vi "AutoThresholdLocalization-4.vi"(4 "[IN] Gauss Filter":bool, 5 "[IN] Method":i32(ring) items=["clustering", "entropy", "metric", "moments", "inter-class variance"], 6 "[IN] Autothreshold Images \nInstead Of Generated U8":bool, 7 "[IN] Median Filter":bool, 8 "error IN":errorcluster, 10 "[IN] Binarized Image":T3, 11 "[IN] Source Image":T3) -> (0 "error OUT":errorcluster, 2 "[OUT] X,Y Coordinates":dbl[](array[numeric]))   [LabVIEW 2020]
uses:
  <vilib>/vision/Image Controls.llb/IMAQ Image.ctl
  <vilib>/vision/Image Controls.llb/IMAQ Rounding Mode.ctl
  <vilib>/vision/NI_Vision_Development_Module.lvlib
panel:
  in  "Selection Values":T2(array[cluster])=[{"Measurement Parameter"=22, "Range Lower Value"=10.0, "Range Upper Value"=800.0, "Range"=FALSE, "Measurement Type"=FALSE}] {"Measurement Parameter" items=["Center of Mass X", "Center of Mass Y", "First Pixel X", "First Pixel Y", "Bounding Rect Left", "Bounding Rect Top", "Bounding Rect Right", "Bounding Rect Bottom", "Max Feret Diameter Start X", "Max Feret Diameter Start Y", "Max Feret Diameter End X", "Max Feret Diameter End Y", "Max Horiz. Segment Length Left", "Max Horiz. Segment Length Right", "Max Horiz. Segment Length Row", "-", "Bounding Rect Width", "Bounding Rect Height", "Bounding Rect Diagonal", "Perimeter", "Convex Hull Perimeter", "Holes' Perimeter", "Max Feret Diameter", "Equivalent Ellipse Major Axis", "Equivalent Ellipse Minor Axis", "Equivalent Ellipse Minor Axis (Feret)", "Equivalent Rect Long Side", "Equivalent Rect Short Side", "Equivalent Rect Diagonal", "Equivalent Rect Short Side (Feret)", "Average Horiz. Segment Length", "Average Vert. Segment Length", "Hydraulic Radius", "Waddel Disk Diameter", "-", "Area", "Holes' Area", "Particle & Holes' Area", "Convex Hull Area", "Image Area", "-", "Number of Holes", "Number of Horiz. Segments", "Number of Vert. Segments", "-", "Orientation", "Max Feret Diameter Orientation", "-", "% Area/Image Area", "% Area/(Particle & Holes' Area)", "Ratio of Equivalent Ellipse Axes", "Ratio of Equivalent Rect Sides", "-", "Elongation Factor", "Compactness Factor", "Heywood Circularity Factor", "Type Factor", "-", "Sum X", "Sum Y", "Sum XX", "Sum XY", "Sum YY", "Sum XXX", "Sum XXY", "Sum XYY", "Sum YYY", "-", "Moment of Inertia XX", "Moment of Inertia XY", "Moment of Inertia YY", "Moment of Inertia XXX", "Moment of Inertia XXY", "Moment of Inertia XYY", "Moment of Inertia YYY", "Norm. Moment of Inertia XX", "Norm. Moment of Inertia XY", "Norm. Moment of Inertia YY", "Norm. Moment of Inertia XXX", "Norm. Moment of Inertia XXY", "Norm. Moment of Inertia XYY", "Norm. Moment of Inertia YYY", "Hu Moment 1", "Hu Moment 2", "Hu Moment 3", "Hu Moment 4", "Hu Moment 5", "Hu Moment 6", "Hu Moment 7"]}
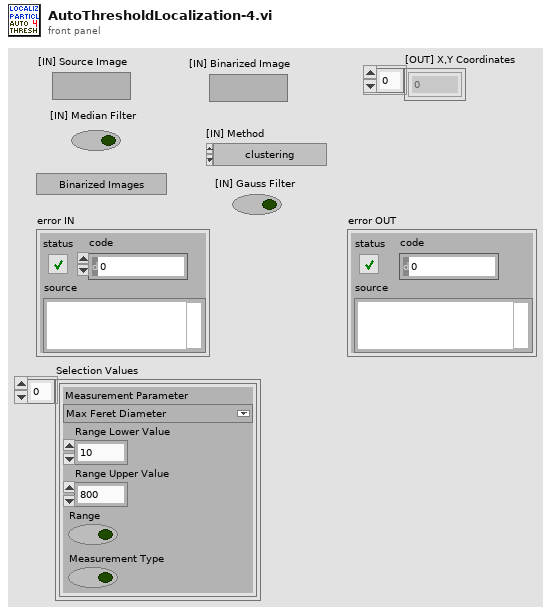
[diagram p1: front panel]
types:
  T1 = typedef "Particle Parameters" = i32
  T2 = cluster{"Measurement Parameter":T1, "Range Lower Value":dbl, "Range Upper Value":dbl, "Range":bool, "Measurement Type":bool}[]
  T3 = typedef "IMAQ Image.ctl" = refnum<image>
  T4 = typedef "Image Type" = u32
  T5 = cluster{"X Size":i32, "Y Size":i32, "Order #":i32}
  T6 = typedef "IMAQ Rounding Mode.ctl" = enum16{"Optimize", "Truncate"}
  T7 = cluster{"Area":dbl, "Number of Holes":dbl, "Bounding Rect":cluster{"Left":dbl, "Top":dbl, "Right":dbl, "Bottom":dbl}, "Center of Mass":cluster{"X":dbl, "Y":dbl}, "Orientation":dbl, "Dimensions":cluster{"Width":dbl, "Height":dbl}}[]
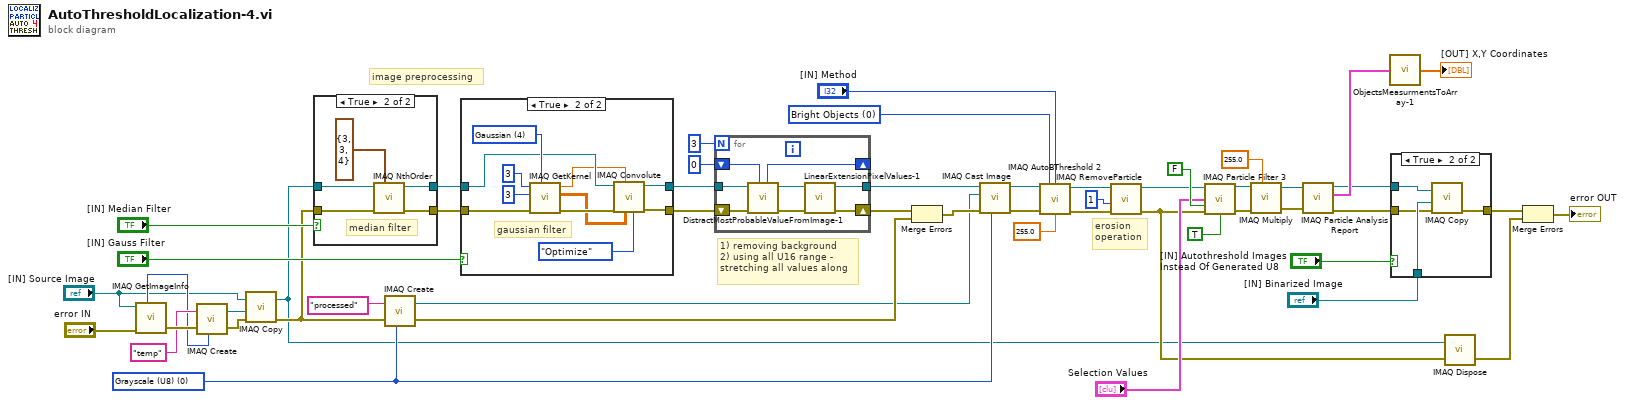
[diagram p0: block diagram]
diagram:
  w42 = u32 0 items=["Bright Objects", "Dark Objects"] ("Look For (Bright Objects)")
  w27 = T4 0 items=["Grayscale (U8)", "Grayscale (I16)", "Grayscale (SGL)", "Complex (CSG)", "RGB (U32)", "HSL (U32)", "RGB (U64)", "Grayscale (U16)"] ("Image Type")
  # "erosion\noperation"
  # "1) removing background\n2) using all U16 range - \nstretching all values along"
  # "image preprocessing"
  n1 = call "IMAQ GetImageInfo"("error in (no error)"="error IN", "Image"="[IN] Source Image") -> ("error out"=w12:errorcluster, "Image Type"=w10:T4)  [unwired: 2 in, 6 out]
  n2 = call "IMAQ Create"("Image Name"="temp", "Image Type"=w10, "error in (no error)"=w12) -> ("New Image"=w8:T3, "error out"=w9:errorcluster)  [unwired: 2 in]
  n3 = call "IMAQ Copy"("error in (no error)"=w9, "Image Dst"=w8, "Image Src"="[IN] Source Image") -> ("error out"=w6:errorcluster, "Image Dst Out"=w4:T3)  [unwired: 3 in]
  n4 = case shown="True" "[IN] Median Filter" {
    tunnel: w4 -> [w53 w57]
    tunnel: w6 -> [w52 w56]
    tunnel: [w53 w55] -> w18
    tunnel: [w52 w54] -> w17
    frame False {
    }
    frame True {
      # "median filter"
      n5 = call "IMAQ NthOrder"("Image Src"=w57, "Size & Order #"=T5 {"X Size"=3, "Y Size"=3, "Order #"=4}, "error in (no error)"=w56) -> ("Image Dst Out"=w55:T3, "error out"=w54:errorcluster)  [unwired: 4 in]
    }
  }
  n6 = call "IMAQ Create"("Image Name"="processed", "Image Type"=w27, "error in (no error)"=w6) -> ("New Image"=w23:T3, "error out"=w25:errorcluster)  [unwired: 2 in]
  n7 = case shown="True" "[IN] Gauss Filter" {
    tunnel: w18 -> [w60 w66]
    tunnel: w17 -> [w59 w68]
    tunnel: [w60 w63] -> w16
    tunnel: [w59 w62] -> w15
    frame False {
    }
    frame True {
      w69 = u16 4 items=["Gradient"=1, "Laplacian"=2, "Smoothing"=3, "Gaussian"=4] ("Kernel Family")
      # "gaussian filter"
      n8 = call "IMAQ GetKernel"("Kernel Family"=w69, "error in (no error)"=w68, "Kernel Number"=3, "Kernel Size (3,5,...)"=3) -> ("error out"=w67:errorcluster, "Kernel"=w64:sgl[][], "Divider"=w65:sgl)  [unwired: 4 in, 1 out]
      n9 = call "IMAQ Convolute"("Rounding Mode"=IMAQ_Rounding_Mode."Optimize", "Kernel"=w64, "Divider (kernel sum)"=w65, "error in (no error)"=w67, "Image Src"=w66) -> ("error out"=w62:errorcluster, "Image Dst Out"=w63:T3)  [unwired: 5 in]
    }
  }
  n10 = for {
    N: 3 -> [_]
    shift-right: [w73] -> w26
    shift-left: w15 -> [w77]
    shift-right: [w72] -> _
    shift-left: 0 ("[IN] # Iteration") -> [w79]
    tunnel: w16 -> [w78]
    tunnel: [w74] -> w46
    n11 = call "DistractMostProbableValueFromImage-1.vi"("[IN] # Iteration"=w79, "error in"=w77, "[IN] Max Projected Image"=w78) -> ("error out"=w75:errorcluster, "[OUT] Processed Image"=w76:T3, "[OUT] # Iteration"=w72:i32)  [unwired: 6 in]
    n12 = call "LinearExtensionPixelValues-1.vi"("error in"=w75, "[IN] Max Projected Image"=w76) -> ("error out"=w73:errorcluster, "[OUT] Processed Image"=w74:T3)  [unwired: 8 in]
  }
  n13 = Merge Errors(w26, w25) -> (w24:errorcluster)
  n14 = call "IMAQ Cast Image"("Image Type"=w27, "error in (no error)"=w24, "Image Dst"=w23, "Image Src"=w46) -> ("error out"=w44:errorcluster, "Image Dst Out"=w45:T3)  [unwired: 6 in]
  n15 = call "IMAQ AutoBThreshold 2"("Image Src"=w45, "Look For (Bright Objects)"=w42, "Method (clustering)"="[IN] Method", "error in (no error)"=w44, "Replace Value (1)"=sgl 255.0) -> ("Image Dst Out"=w21:T3, "error out"=w22:errorcluster)  [unwired: 8 in, 1 out]
  n16 = call "IMAQ RemoveParticle"("error in (no error)"=w22, "Number of Erosion"=1, "Image Src"=w21) -> ("error out"=w5:errorcluster, "Image Dst Out"=w19:T3)  [unwired: 7 in]
  n17 = call "IMAQ Particle Filter 3"("Image Src"=w19, "Selection Values"="Selection Values", "Keep/Remove Particles (F)"=FALSE, "error in (no error)"=w5, "Fill Holes? (F)"=TRUE ("Connectivity 4/8 (8)")) -> ("Image Dst Out"=w36:T3, "error out"=w37:errorcluster)  [unwired: 8 in, 1 out]
  n18 = call "IMAQ Multiply"("Image Src A"=w36, "Constant"=255.0, "error in (no error)"=w37) -> ("Image Dst Out"=w35:T3, "error out"=w34:errorcluster)  [unwired: 4 in]
  n19 = call "IMAQ Particle Analysis Report"("error in (no error)"=w34, "Image"=w35) -> ("error out"=w31:errorcluster, "Particle Reports (Pixels)"=w32:T7, "Image Out (duplicate)"=w30:T3)  [unwired: 4 in, 3 out]
  n20 = call "ObjectsMeasurmentsToArray-1.vi"("[IN] Particle Reports (Pixels)"=w32) -> ("[OUT] X,Y Coordinates"=→"[OUT] X,Y Coordinates":dbl[])
  n21 = case shown="True" "[IN] Autothreshold Images \nInstead Of Generated U8" {
    tunnel: w31 -> [w80 w82]
    tunnel: [w80 w84] -> w2
    tunnel: w30 -> [_ w81]
    tunnel: "[IN] Binarized Image" -> [_ w83]
    frame False {
    }
    frame True {
      n22 = call "IMAQ Copy"("error in (no error)"=w82, "Image Dst"=w83, "Image Src"=w81) -> ("error out"=w84:errorcluster)  [unwired: 3 in, 1 out]
    }
  }
  n23 = call "IMAQ Dispose"("Image"=w4, "error in (no error)"=w5) -> ("error out"=w3:errorcluster)  [unwired: 4 in]
  n24 = Merge Errors(w2, w3) -> (→"error OUT":errorcluster)
